vi "ADC Code Histogram.vi"(8 "error in (no error)":errorcluster, 10 "number of bits":i32, 11 "codes":i32[](array[numeric])) -> (0 "error out":errorcluster, 3 "histogram":T1)   [LabVIEW 2021]
uses:
  <vilib>/Analysis/1siggen.llb/Ramp Pattern by Samples.vi
  <vilib>/Analysis/NI_AALBase.lvlib
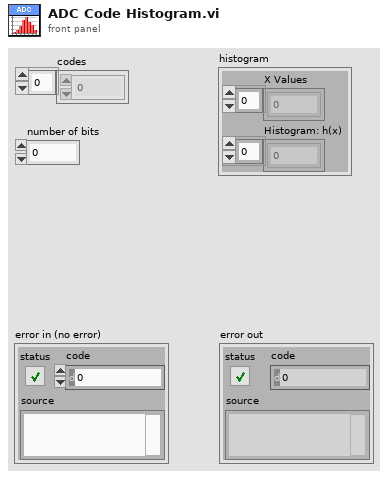
[diagram p1: front panel]
types:
  T1 = cluster{"X Values":dbl[], "Histogram: h(x)":i32[]}
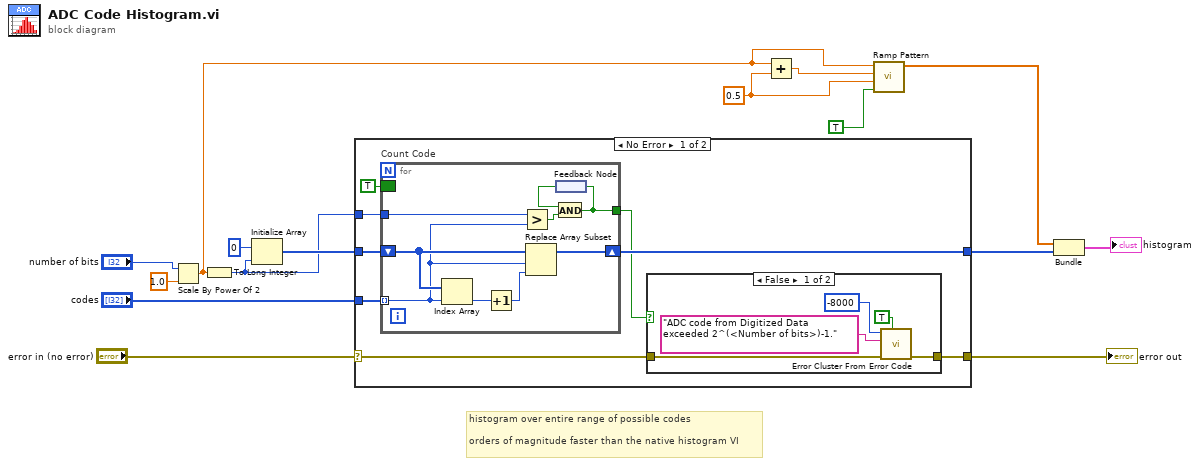
[diagram p0: block diagram]
diagram:
  w5 = 0.5 ("start")
  # "histogram over entire range of possible codes\n\norders of magnitude faster than the native histogram VI"
  n1 = Scale By Power Of 2(n="number of bits", x=1.0) -> (x*2^n=w3:dbl)
  n2 = To Long Integer(number=w3) -> (32bit integer=w11:i32)
  n3 = Initialize Array(u32 0 ("element"), w11) -> (w15:u32[])
  n4 = case shown="No Error" "error in (no error)" {
    selector: "error in (no error)" -> [w17 w39]
    tunnel: "codes" -> [w23 _]
    tunnel: [w21 _] -> w7
    tunnel: [w18 w39] -> w8
    tunnel: w15 -> [w22 _]
    tunnel: w11 -> [w20 _]
    frame No Error {
      n5 = for "Count Code" {
        tunnel: w23 -> [w30] mode=indexing
        shift-right: [w38] -> w21
        shift-left: w22 -> [w37]
        tunnel: w20 -> [w35]
        border: TRUE -> [_]
        tunnel: [w31] -> w16
        n6 = Index Array(array=w37, index=w30) -> (element=w36:u32)
        n7 = Increment(x=w36) -> (x+1=w34:u32)
        n8 = Greater?(x=w35, y=w30) -> (0:w33:bool)
        n9 = Replace Array Subset(array=w37, new element=w34, index=w30) -> (w38:u32[])
        n10 = feedback #1() -> (w32:bool)
        n11 = And(x=w32, y=w33) -> (x .and. y?=w31:bool)
        n12 = feedback-in #1(w31) -> ()
      }
      n13 = case shown="False" w16 {
        tunnel: [w28 w29] -> w18
        tunnel: w17 -> [w27 w29]
        frame False {
          n14 = call <vilib>:"Error Cluster From Error Code.vi"("show call chain? (False)"=TRUE, "error in (no error)"=w27, "error message (\"\")"="ADC code from Digitized Data exceeded 2^(<Number of bits>)-1." ("error message (\"\")"), "error code (0)"=-8000) -> ("error out"=w28:errorcluster)  [unwired: 5 in]
        }
        frame True {
        }
      }
    }
    frame Error {
    }
  }
  "error out" <- w8
  n15 = Add(x=w3, y=w5) -> (x+y=w4:dbl)
  n16 = call-poly <vilib>:"Ramp Pattern.vi"("exclude end?"=TRUE, "start"=w5, "end"=w4, "samples"=w3) -> ("Ramp Pattern"=w2:dbl[])  [unwired: 6 in, 1 out]
  n17 = Bundle("Ramp Pattern"=w2, w7) -> (→"histogram":cluster{"Ramp Pattern":dbl[], u32[]})  [unwired: 1 out]
